vi "write_timing_array.vi"(4 "error in":errorcluster, 5 "delay array":dbl[](array[numeric]), 6 "time unit":enum16{"s", "ms", "us", "ns"}(ring), 7 "VISA resource in":refnum<visa-resource-name>) -> (0 "error out 2":errorcluster, 3 "VISA resource out":refnum<visa-resource-name>)   [LabVIEW 2011]
doc: "Reads all delay values stored in the DG645 and returns them in an array, from t0 to H.\nSee DG645 documentation for mor info."
panel:
  out "Array":string[](array[string])
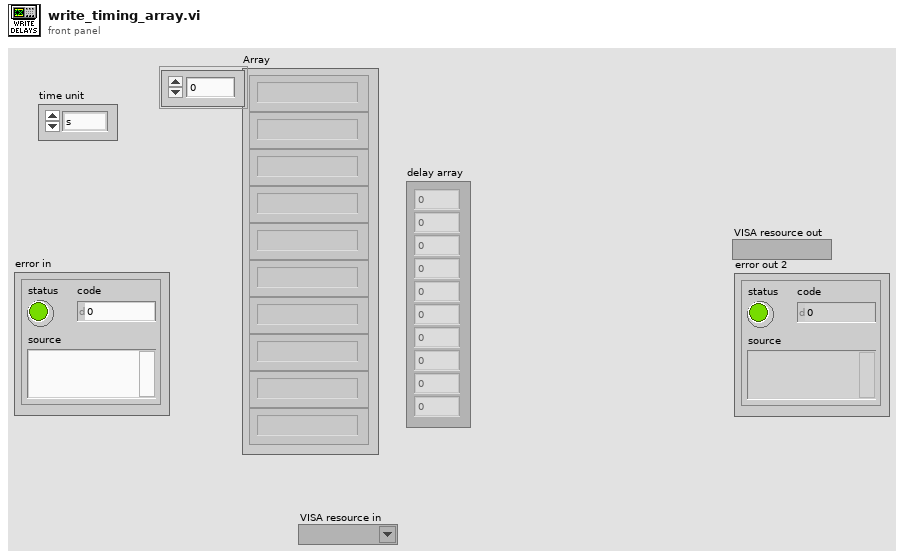
[diagram p1: front panel]
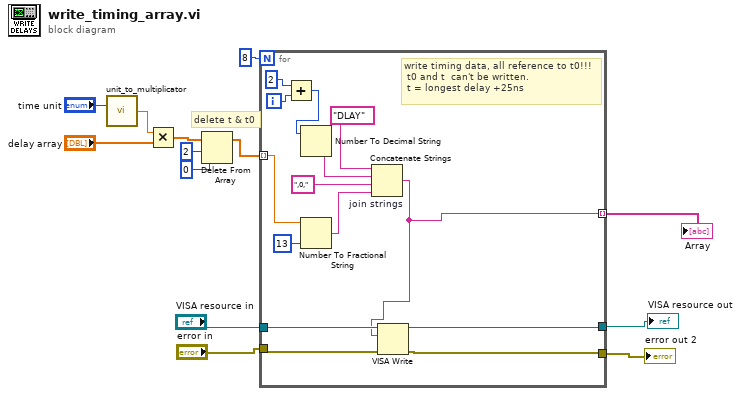
[diagram p0: block diagram]
diagram:
  # "delete t & t0"
  n1 = call "unit_to_multiplicator.vi"("time unit"="time unit") -> ("multiplicator"=w4:dbl)
  n2 = Multiply(x=w4, y="delay array") -> (x*y=w1:dbl[])
  n3 = Delete From Array(array=w1, length=2, index=0) -> (array with subset deleted=w5:dbl[])  [unwired: 1 out]
  n4 = for {
    N: 8 -> [_]
    tunnel: "error in" -> [w25]
    tunnel: [w26] -> w9
    tunnel: "VISA resource in" -> [w22]
    tunnel: [w27] -> w10
    tunnel: [w18] -> w8 mode=indexing
    tunnel: w5 -> [w17] mode=indexing
    i -> [w20]
    # "write timing data, all reference to t0!!!\n t0 and t  can't be written.\n t = longest delay +25ns"
    n5 = Add(x=2, y=w20) -> (x+y=w15:i32)
    n6 = Number To Decimal String(number=w15) -> (decimal integer string=w23:string)  [unwired: 1 in]
    n7 = Number To Fractional String(number=w17, precision (6)=i16 13) -> (F-format string=w19:string)  [unwired: 2 in]
    n8 = Concatenate Strings "join strings"("DLAY" ("string"), w23, ",0," ("string"), w19) -> (w18:string)
    n9 = VISA Write(VISA resource name=w22, write buffer=w18, error in (no error)=w25) -> (VISA resource name out=w27:refnum<visa-resource-name>, error out=w26:errorcluster)  [unwired: 1 out]
  }
  "VISA resource out" <- w10
  "error out 2" <- w9
  "Array" <- w8
